vi "RSZVB Get Power Stimulus.vi"(8 "error in (no error)":errorcluster {"code" format="%.0x"}, 10 "Channel (1)":i32=1, 11 "VISA session":refnum<visa-resource-name>) -> (0 "error out":errorcluster {"code" format="%.0x"}, 1 "Power Stimulus":string, 3 "dup VISA session":refnum<visa-resource-name>)   [LabVIEW 2011]
doc: "This VI returns the stimulus signal that is used for the definition of the power sweep range or fixed power. \n\nNote(s):\n\n(1) This command is particularly useful in arbitrary mode (with option R&S ZVA-K4), where the frequencies and source powers at the ports are independent. \n\n(2) For R&S ZVA and ZVT analyzers without option R&S ZVA-K4, all powers are coupled so that this selection has no effect. \n\n(3) For R&S ZVB analyzers, all frequencies are coupled so that this selection has no effect. \n\nRemote-control command(s):\n[SENSe<Ch>:]SWEep:AXIS:POWer?"
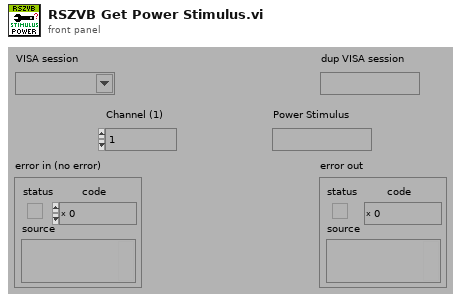
[diagram p1: front panel]
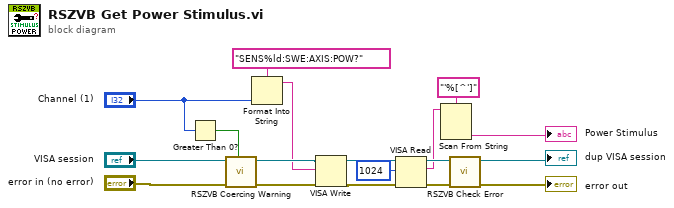
[diagram p0: block diagram]
diagram:
  n1 = Greater Than 0?(x="Channel (1)") -> (x > 0?=w10:bool)
  n2 = call "RSZVB Coercing Warning.vi"("In Range?"=w10, "error in (no error)"="error in (no error)", "VISA session"="VISA session") -> ("error out"=w8:errorcluster, "dup VISA session"=w9:refnum<visa-resource-name>)  [unwired: 7 in]
  n3 = Format Into String(format string="SENS%ld:SWE:AXIS:POW?", "Channel (1)") -> (resulting string=w7:string)  [unwired: 2 in, 1 out]
  n4 = VISA Write(VISA resource name=w9, write buffer=w7, error in (no error)=w8) -> (VISA resource name out=w15:refnum<visa-resource-name>, error out=w14:errorcluster)  [unwired: 1 out]
  n5 = VISA Read(VISA resource name=w15, byte count=u32 1024 ("byte count (0)"), error in (no error)=w14) -> (VISA resource name out=w18:refnum<visa-resource-name>, read buffer=w12:string, error out=w17:errorcluster)  [unwired: 1 out]
  n6 = Scan From String(format string="'%[^']", input string=w12) -> (output 1=→"Power Stimulus":string)  [unwired: 3 in, 3 out]
  n7 = call "RSZVB Check Error.vi"("error in (no error)"=w17, "VISA session"=w18) -> ("error out"=→"error out":errorcluster, "dup VISA session"=→"dup VISA session":refnum<visa-resource-name>)  [unwired: 8 in]
